vi "MainClose Queue.vi"(8 "error in":errorcluster) -> (0 "error out":errorcluster)   [LabVIEW 2022 SP3]
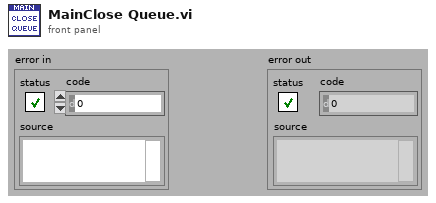
[diagram p1: front panel]
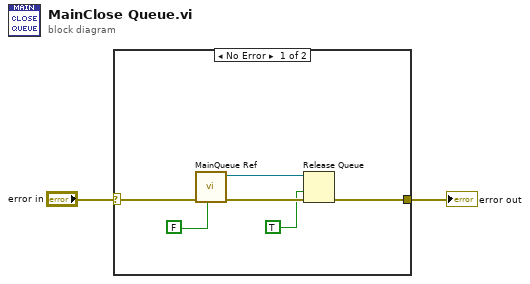
[diagram p0: block diagram]
diagram:
  n1 = case shown="No Error" "error in" {
    selector: "error in" -> [w7 w9]
    tunnel: [w8 w9] -> w1
    frame No Error {
      n2 = call "MainQueue Ref.vi"("Write:T/Read:(F)"=FALSE, "error in"=w7) -> ("error out"=w6:errorcluster, "queue out"=w5:refnum<queue>)  [unwired: 8 in]
      n3 = Release Queue(queue=w5, force destroy? (F)=TRUE, error in (no error)=w6) -> (error out=w8:errorcluster)  [unwired: 2 out]
    }
    frame Error {
    }
  }
  "error out" <- w1
